vi "Configure Basic IMDistortion.vi"(7 "Append Traces (T: Enable)":bool=TRUE, 8 "error in (no error)":errorcluster, 9 "Product Selection (0: imdSMPTE2)":i32(ring) items=["imdSMPTE2", "imdSMPTE23", "imdSMPTE234"], 10 "Waveform (0: wiSMPTE)":i32(ring) items=["wiSMPTE", "wiCCIF", "wiDIM"], 11 "VISA resource name":refnum<visa-resource-name>) -> (0 "error out":errorcluster, 3 "VISA resource name out":refnum<visa-resource-name>)   [LabVIEW 2014, in "Stanford Research SR1.lvlib"]
doc: "Configures the basic attributes of the IMDistortion Quick Measurement."
uses:
  Stanford Research SR1.lvlib
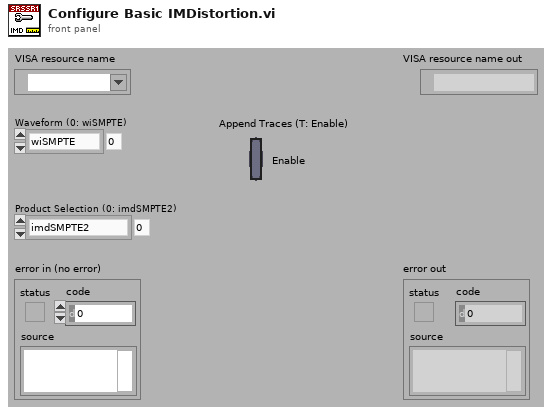
[diagram p1: front panel]
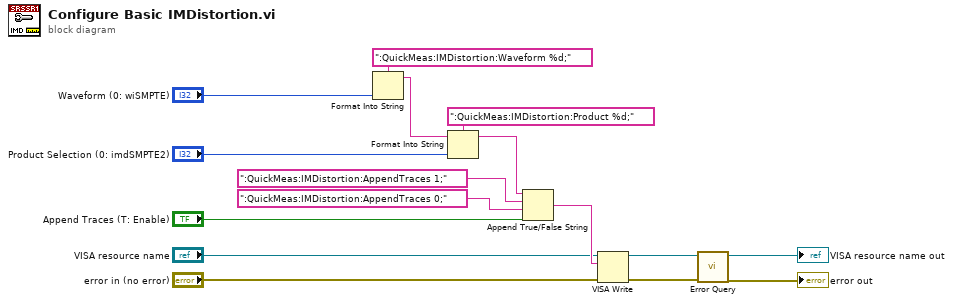
[diagram p0: block diagram]
diagram:
  n1 = Format Into String(format string=":QuickMeas:IMDistortion:Waveform %d;", "Waveform (0: wiSMPTE)") -> (resulting string=w14:string)  [unwired: 2 in, 1 out]
  n2 = Format Into String(format string=":QuickMeas:IMDistortion:Product %d;", initial string=w14, "Product Selection (0: imdSMPTE2)") -> (resulting string=w11:string)  [unwired: 1 in, 1 out]
  n3 = Append True/False String(1:"Append Traces (T: Enable)", 2:":QuickMeas:IMDistortion:AppendTraces 0;", 3:":QuickMeas:IMDistortion:AppendTraces 1;", 4:w11) -> (0:w7:string)
  n4 = VISA Write(VISA resource name="VISA resource name", write buffer=w7, error in (no error)="error in (no error)") -> (VISA resource name out=w4:refnum<visa-resource-name>, error out=w3:errorcluster)  [unwired: 1 out]
  n5 = call "Error Query.vi"("error in (no error)"=w3, "VISA resource name"=w4) -> ("error out"=→"error out":errorcluster, "VISA resource name out"=→"VISA resource name out":refnum<visa-resource-name>)  [unwired: 6 in, 2 out]
